vi "LEP_RV_CreateUVProject.vi"(8 "error in (no error)":errorcluster, 9 "Build Path":path=path "c:/tmp/test", 10 "Target":string="Build Spec Name") -> (0 "error out":errorcluster)   [LabVIEW 2011]
doc: "Runs the embedded application on a console located in the <B>Build Path</B> directory ."
panel:
  in  "Force Update (not implemented yet)":bool
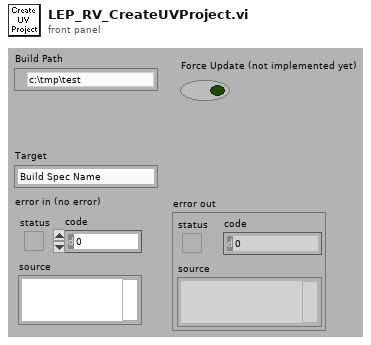
[diagram p1: front panel]
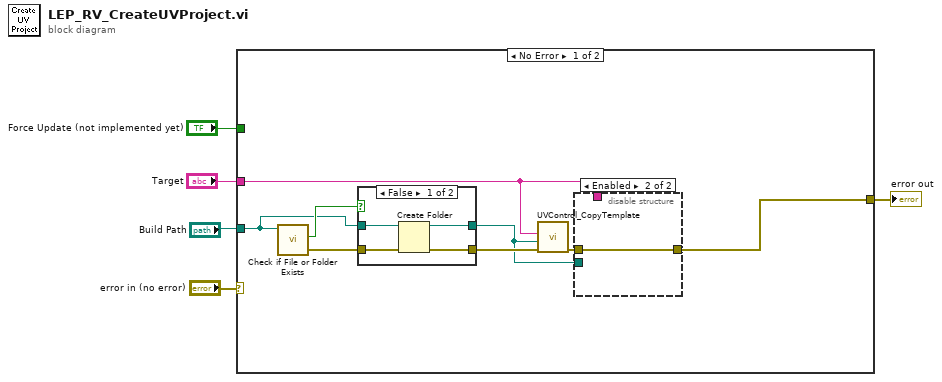
[diagram p0: block diagram]
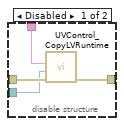
[diagram p2: hidden frame]
diagram:
  n1 = case shown="No Error" "error in (no error)" {
    selector: "error in (no error)" -> [_ w25]
    tunnel: "Build Path" -> [w8 _]
    tunnel: [w12 w25] -> w3
    tunnel: "Force Update (not implemented yet)" -> [_ _]
    tunnel: "Target" -> [w6 _]
    frame No Error {
      n2 = call <vilib>:"Check if File or Folder Exists.vi"("path"=w8) -> ("error out"=w13:errorcluster, "file or folder exists?"=w9:bool)  [unwired: 8 in, 1 out]
      n3 = case shown="False" w9 {
        tunnel: w13 -> [w22 w23]
        tunnel: w8 -> [w21 w24]
        tunnel: [w20 w24] -> w7
        tunnel: [w19 w23] -> w11
        frame False {
          n4 = Create Folder(path (use dialog)=w21, error in=w22) -> (created path=w20:path, error out=w19:errorcluster)  [unwired: 1 in, 1 out]
        }
        frame True {
        }
      }
      n5 = call "UVControl_CopyTemplate.vi"("error in (no error)"=w11, "UV Project Path"=w7, "Target"=w6) -> ("error out"=w10:errorcluster)  [unwired: 8 in]
      n6 = disable-structure shown="Enabled" {
        disable-tunnel: [w17 w18] -> w12
        disable-tunnel: w10 -> [w16 w18]
        disable-tunnel: w7 -> [w15 _]
        disable-tunnel: w6 -> [w14 _]
        frame Disabled {
          n7 = call "UVControl_CopyLVRuntime.vi"("error in (no error)"=w16, "UV Project Path"=w15, "Target"=w14) -> ("error out"=w17:errorcluster)  [unwired: 8 in]
        }
        frame Enabled {
        }
      }
    }
    frame Error {
    }
  }
  "error out" <- w3
